vi "fgv_PXI-5110_data.vi"(7 "cmd":T2, 11 "data":T1={"Waveform(s)"=[], "Actual Record Length"=1000, "Actual Sample Rate"=10000000.0, "Auto Triggered"=FALSE} {"Actual Sample Rate" format="%#.2p"}) -> (3 "data 2":T1={"Waveform(s)"=[], "Actual Record Length"=1000, "Actual Sample Rate"=10000000.0, "Auto Triggered"=FALSE} {"Actual Sample Rate" format="%#.2p"})   [LabVIEW 2021]
uses:
  ctrl/rw.ctl
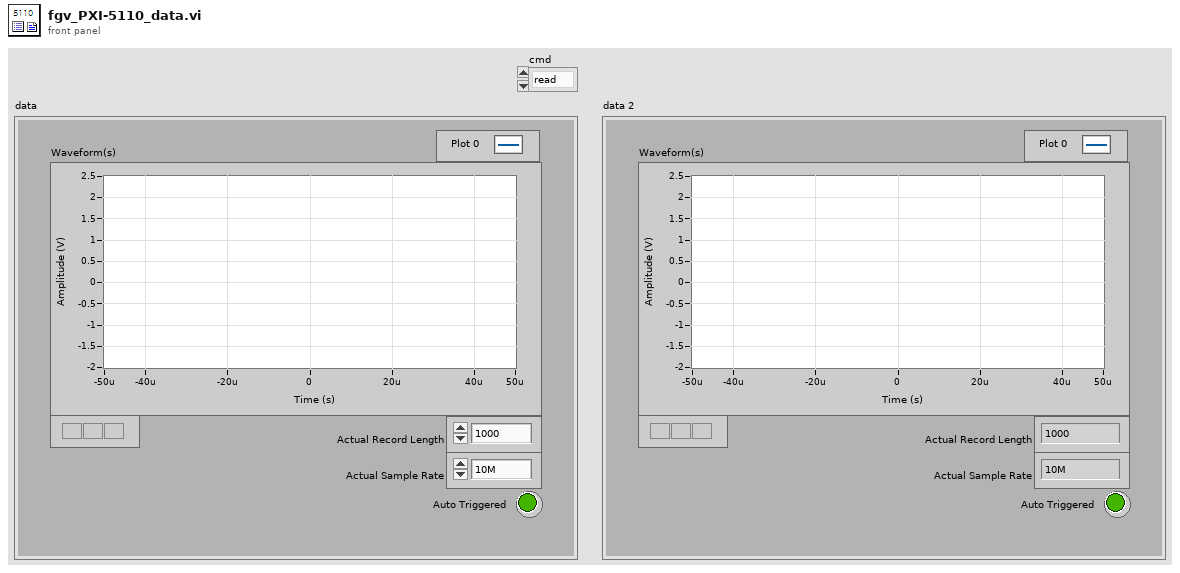
[diagram p1: front panel]
types:
  T1 = cluster{"Waveform(s)":cluster{"relativeInitialX":dbl, "xIncrement":dbl, "wfm":dbl[]}[], "Actual Record Length":i32, "Actual Sample Rate":dbl, "Auto Triggered":bool}
  T2 = typedef "rw.ctl" = enum16{"read", "write"}
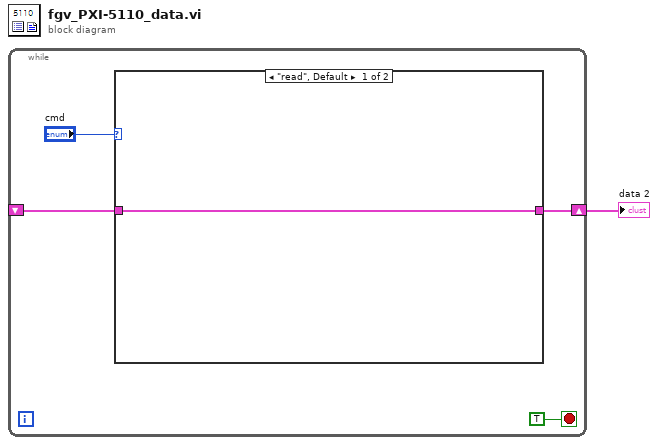
[diagram p0: block diagram]
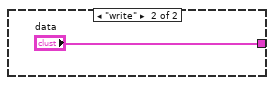
[diagram p2: hidden frame]
diagram:
  n1 = while {
    shift-right: [w3] -> w1
    shift-left: _ -> [w2]
    stop <- TRUE stop-if-true
    n2 = case shown="\"read\", Default" "cmd" {
      tunnel: [w6 "data"] -> w3
      tunnel: w2 -> [w6 _]
      frame "read", Default {
      }
      frame "write" {
      }
    }
  }
  "data 2" <- w1
